vi "Do.vi"(8 "error in (no error)":errorcluster, 10 "Actor in":refnum<class "Actor.lvclass">, 11 "Launch GUI Msg":refnum<class "Launch GUI Msg.lvclass">) -> (0 "error out":errorcluster, 2 "Actor out":refnum<class "Actor.lvclass">)   [LabVIEW 2012, in "CS++BaseActor.lvlib" / "Launch GUI Msg.lvclass"]
doc: "This VI delivers the message to the actor by calling the appropriate method(s) on the actor."
uses:
  Launch GUI Msg.lvclass
  CS++BaseActor/CS++BaseActor.lvclass
  <vilib>/ActorFramework/Actor/Actor.lvclass
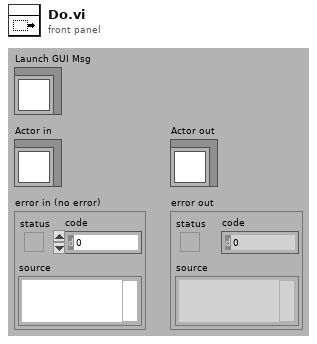
[diagram p1: front panel]
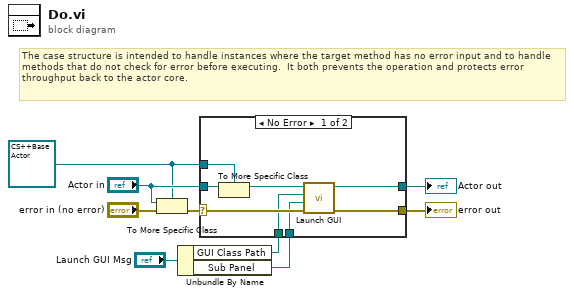
[diagram p0: block diagram]
diagram:
  w1 = refnum<class "CS++BaseActor.lvclass"> refnum ("CS++BaseActor.lvlib:CS++BaseActor.lvclass")
  # "The case structure is intended to handle instances where the target method has no error input and to handle methods that do not check for error before executing.  It both prevents the operation and protects error throughput back to the actor core."
  n1 = To More Specific Class(target class=w1, reference="Actor in", error in="error in (no error)") -> (error out=w8:errorcluster)  [unwired: 1 out]
  n2 = Unbundle By Name("Launch GUI Msg") -> ("GUI Class Path"=w3:path, "Sub Panel"=w2:refnum<vi>)
  n3 = case shown="No Error" w8 {
    selector: w8 -> [w15 w19]
    tunnel: [w17 w19] -> w7
    tunnel: [w16 w18] -> w6
    tunnel: "Actor in" -> [w14 w18]
    tunnel: w1 -> [w13 _]
    tunnel: w3 -> [w11 _]
    tunnel: w2 -> [w10 _]
    frame No Error {
      n4 = To More Specific Class(target class=w13, reference=w14) -> (specific class reference=w12:refnum<class "CS++BaseActor.lvclass">)  [unwired: 1 in, 1 out]
      n5 = call "Launch GUI.vi"("error in (no error)"=w15, "Sub Panel"=w10, "GUI Class Path"=w11, "CS++BaseActor"=w12) -> ("error out"=w17:errorcluster, "CS++BaseActor"=w16:refnum<class "CS++BaseActor.lvclass">)  [unwired: 6 in]
    }
    frame Error {
      # "If type check fails, pass the original object out again."
    }
  }
  "error out" <- w7
  "Actor out" <- w6
